vi "Set Engine.vi"(8 "error in (no error)":errorcluster, 10 "TSnax:Engine":refnum<class "Engine.lvclass">, 11 "SequenceViewPanel in":refnum<class "SequenceViewPanel.lvclass">) -> (0 "error out":errorcluster, 3 "SequenceViewPanel out":refnum<class "SequenceViewPanel.lvclass">)   [LabVIEW 2020, in "TSnax UI.lvlib" / "SequenceViewPanel.lvclass"]
uses:
  SequenceViewPanel.lvclass
  TSnax/Engine/Engine.lvclass
  SequenceViewPanel.lvclass/SequenceViewPanel.ctl
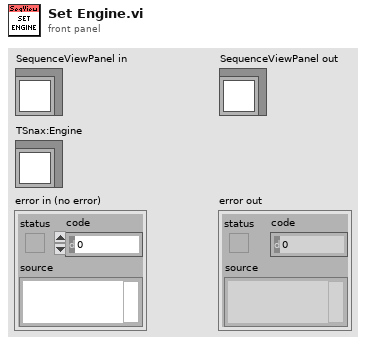
[diagram p1: front panel]
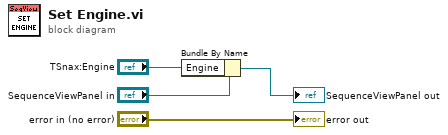
[diagram p0: block diagram]
diagram:
  n1 = Bundle By Name(cluster="SequenceViewPanel in", "Engine"="TSnax:Engine") -> (→"SequenceViewPanel out":refnum<class "SequenceViewPanel.lvclass">)
  "error out" <- "error in (no error)"
